vi "CRYSet Format Text Front Panel.vi"(11 "Vi Ref":refnum<vi>) -> ()   [LabVIEW 2013]
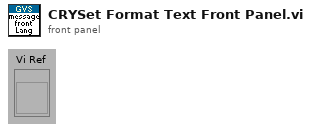
[diagram p1: front panel]
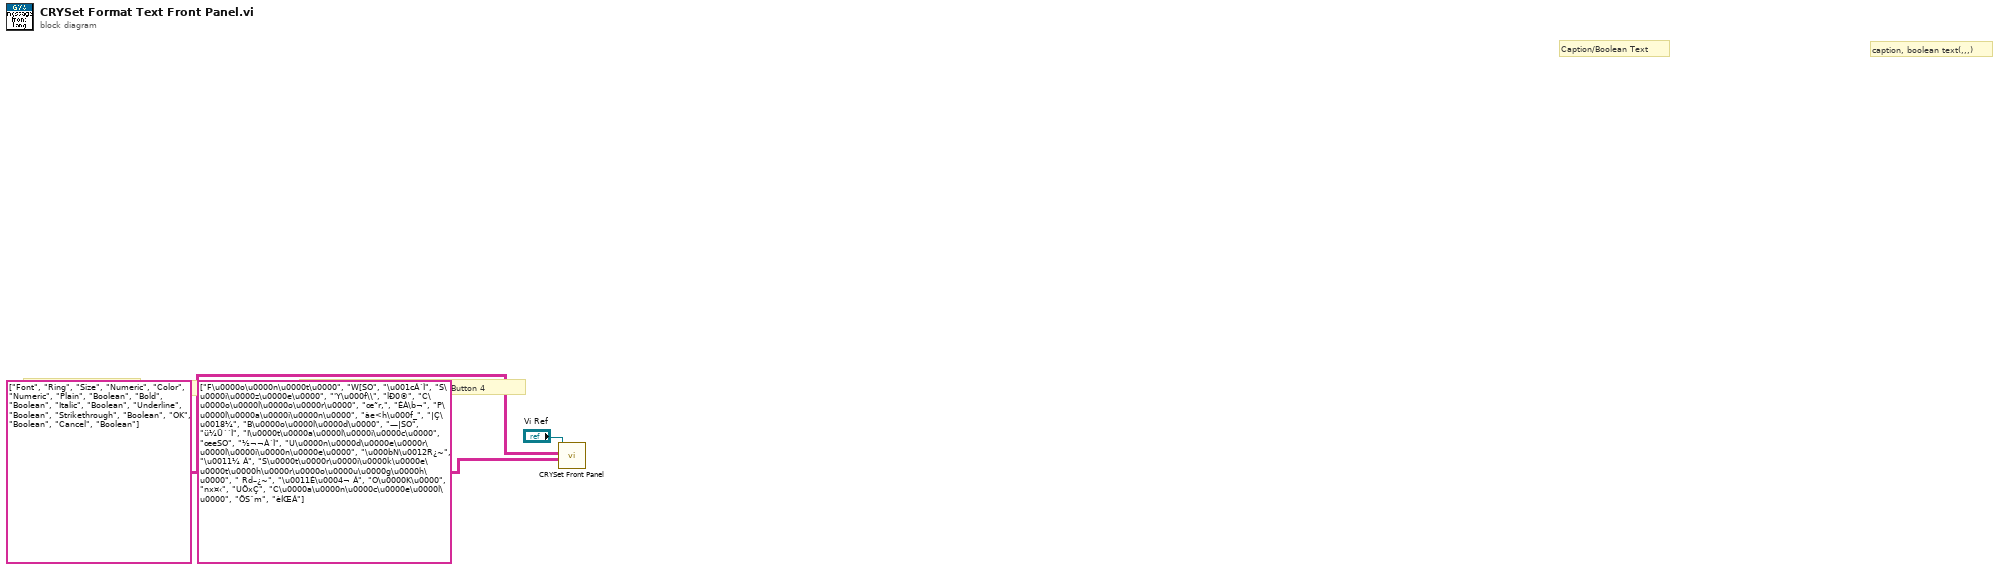
[diagram p0: block diagram]
diagram:
  # "Caption, Tab Page, Multilist Header, Button 4"
  # "Control Type"
  # "Control Name and Tab"
  # "caption, boolean text(,,,)"
  # "Caption/Boolean Text"
  n1 = call "CRYSet Front Panel.vi"("Caption(Boolean Text)"=string[][] [["F\u0000o\u0000n\u0000t\u0000", "W[SO", "\u001cÁ´Ì"], ["S\u0000i\u0000z\u0000e\u0000", "'Y\u000f\\", "lÐ0®"], ["C\u0000o\u0000l\u0000o\u0000r\u0000", "œ˜r‚", "ÉÀ\b¬"], ["P\u0000l\u0000a\u0000i\u0000n\u0000", "àe<h\u000f_", "|Ç\u0018¼"], ["B\u0000o\u0000l\u0000d\u0000", "—|SO", "ü¼Ü´´Ì"], ["I\u0000t\u0000a\u0000l\u0000i\u0000c\u0000", "œeSO", "½¬¬À´Ì"], ["U\u0000n\u0000d\u0000e\u0000r\u0000l\u0000i\u0000n\u0000e\u0000", "\u000bN\u0012R¿~", "\u0011¼ Á"], ["S\u0000t\u0000r\u0000i\u0000k\u0000e\u0000t\u0000h\u0000r\u0000o\u0000u\u0000g\u0000h\u0000", " Rd–¿~", "\u0011É\u0004¬ Á"], ["O\u0000K\u0000", "nx¤‹", "UÖxÇ"], ["C\u0000a\u0000n\u0000c\u0000e\u0000l\u0000", "ÖSˆm", "èÍŒÁ"]], "Control ID and Type(Label Name, Type)"=string[][] [["Font", "Ring"], ["Size", "Numeric"], ["Color", "Numeric"], ["Plain", "Boolean"], ["Bold", "Boolean"], ["Italic", "Boolean"], ["Underline", "Boolean"], ["Strikethrough", "Boolean"], ["OK", "Boolean"], ["Cancel", "Boolean"]], "Vi Ref"="Vi Ref") -> ()  [unwired: 9 in]
